vi "General_data.vi"() -> (0 "String":string)   [LabVIEW 2018]
uses:
  Instrument_Setup.vi
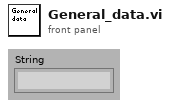
[diagram p1: front panel]
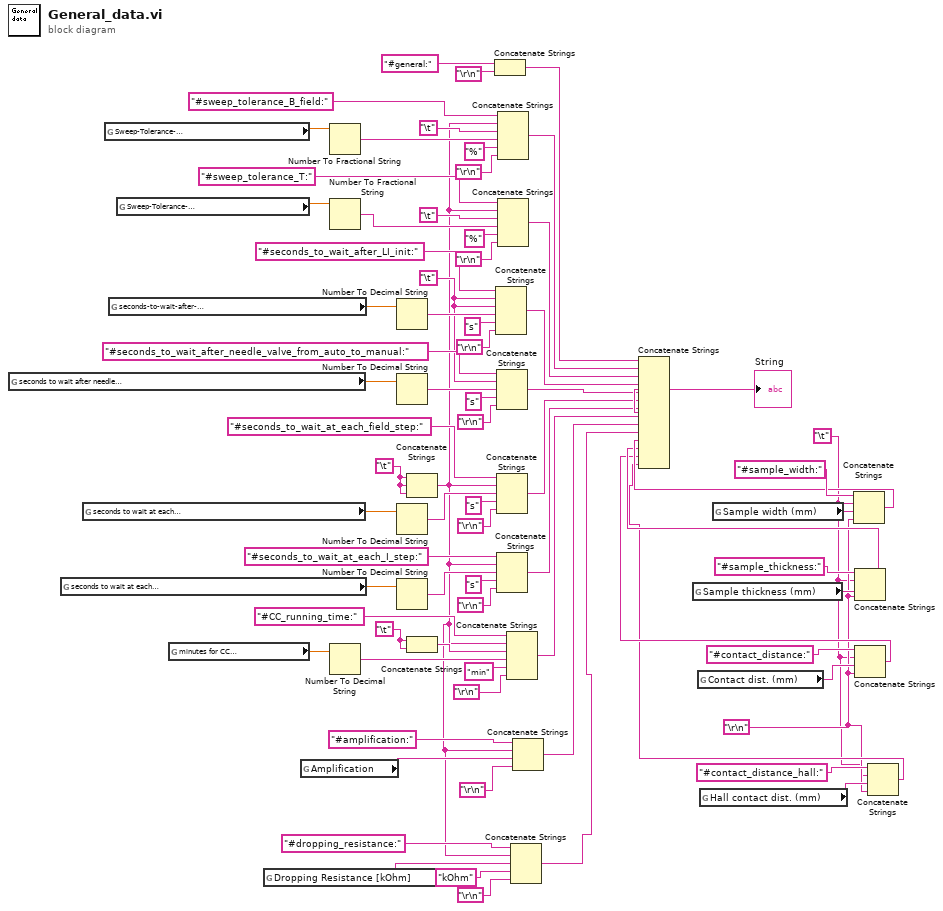
[diagram p0: block diagram]
diagram:
  w2 = "\r\n"
  w1 = "\t"
  w25 = "\t"
  w32 = "\t"
  w33 = "\t"
  n1 = global read "Instrument_Setup.vi" "seconds to wait after needle\nvalve was set from auto to\nmanual"() -> (w53:dbl)
  n2 = global read "Instrument_Setup.vi" "seconds to wait at each\ncurrent step in a I-step sweep"() -> (w65:dbl)
  n3 = global read "Instrument_Setup.vi" "seconds to wait at each\nfield step in a step sweep"() -> (w59:dbl)
  n4 = global read "Instrument_Setup.vi" "Sweep-Tolerance-\nMagnetic-Field"() -> (w35:dbl)
  n5 = global read "Instrument_Setup.vi" "seconds-to-wait-after-\nLock-In-initialization"() -> (w45:dbl)
  n6 = global read "Instrument_Setup.vi" "Sweep-Tolerance-\nTemperature"() -> (w40:dbl)
  n7 = global read "Instrument_Setup.vi" "minutes for CC\nto run"() -> (w68:dbl)
  n8 = global read "Instrument_Setup.vi" "Dropping Resistance [kOhm]"() -> (w19:string)
  n9 = global read "Instrument_Setup.vi" "Amplification"() -> (w23:string)
  n10 = Number To Fractional String(number=w35) -> (F-format string=w36:string)  [unwired: 3 in]
  n11 = Number To Fractional String(number=w40) -> (F-format string=w41:string)  [unwired: 3 in]
  n12 = Number To Decimal String(number=w68) -> (decimal integer string=w52:string)  [unwired: 1 in]
  n13 = Number To Decimal String(number=w45) -> (decimal integer string=w46:string)  [unwired: 1 in]
  n14 = Number To Decimal String(number=w53) -> (decimal integer string=w50:string)  [unwired: 1 in]
  n15 = Number To Decimal String(number=w59) -> (decimal integer string=w57:string)  [unwired: 1 in]
  n16 = Number To Decimal String(number=w65) -> (decimal integer string=w63:string)  [unwired: 1 in]
  n17 = Concatenate Strings(w33, w33, w33) -> (w18:string)
  n18 = Concatenate Strings(w32, w32) -> (w31:string)
  n19 = Concatenate Strings("#general:", "\r\n") -> (w28:string)
  n20 = Concatenate Strings("#seconds_to_wait_after_LI_init:" ("String"), w25, w25, w46, "s" ("String"), "\r\n") -> (w71:string)
  n21 = Concatenate Strings("#seconds_to_wait_after_needle_valve_from_auto_to_manual:" ("String"), w25, w50, "s" ("String"), "\r\n") -> (w72:string)
  n22 = Concatenate Strings("#seconds_to_wait_at_each_field_step:" ("String"), w18, w57, "s" ("String"), "\r\n") -> (w73:string)
  n23 = Concatenate Strings("#seconds_to_wait_at_each_I_step:" ("String"), w18, w63, "s" ("String"), "\r\n") -> (w74:string)
  n24 = Concatenate Strings("#sweep_tolerance_B_field:", w18, "\t", w36, "%" ("String"), "\r\n") -> (w69:string)
  n25 = Concatenate Strings("#sweep_tolerance_T:", w18, "\t", w41, "%" ("String"), "\r\n") -> (w70:string)
  n26 = Concatenate Strings("#CC_running_time:" ("String"), w18, w31, w52, "min" ("String"), "\r\n") -> (w75:string)
  n27 = Concatenate Strings("#dropping_resistance:" ("String"), w18, w19, "kOhm" ("String"), "\r\n") -> (w15:string)
  n28 = Concatenate Strings("#amplification:" ("String"), w18, w23, "\r\n") -> (w21:string)
  n29 = global read "Instrument_Setup.vi" "Sample thickness (mm)"() -> (w11:string)
  n30 = global read "Instrument_Setup.vi" "Contact dist. (mm)"() -> (w10:string)
  n31 = global read "Instrument_Setup.vi" "Hall contact dist. (mm)"() -> (w5:string)
  n32 = global read "Instrument_Setup.vi" "Sample width (mm)"() -> (w12:string)
  n33 = Concatenate Strings("#sample_width:" ("String"), w1, w12, w2) -> (w8:string)
  n34 = Concatenate Strings("#sample_thickness:" ("String"), w1, w11, w2) -> (w7:string)
  n35 = Concatenate Strings("#contact_distance:" ("String"), w1, w10, w2) -> (w6:string)
  n36 = Concatenate Strings("#contact_distance_hall:" ("String"), w1, w5, w2) -> (w3:string)
  n37 = Concatenate Strings(w28, w69, w70, w71, w72, w73, w74, w75, w21, w15, w8, w7, w6, w3) -> (→"String":string)
